vi "KB-SplitRoi TO Recntage.vi"(11 "String 2":string) -> (3 "数组":string[](array[string]))   [LabVIEW 2015]
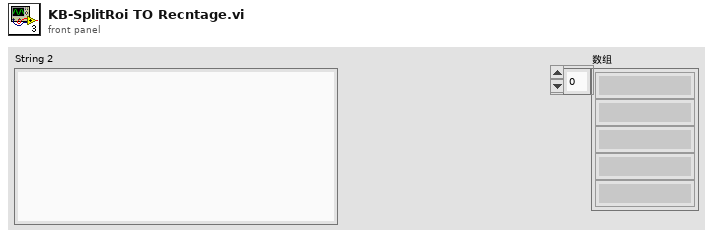
[diagram p1: front panel]
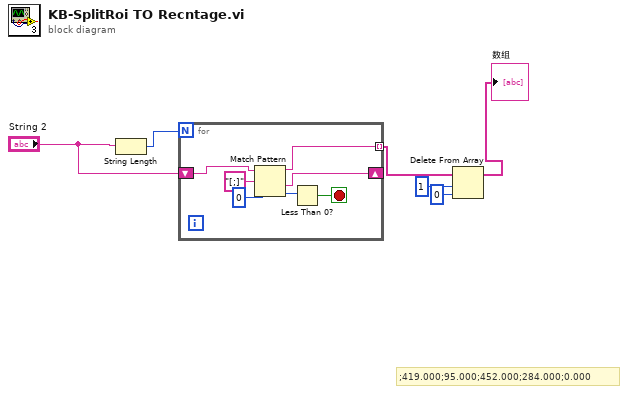
[diagram p0: block diagram]
diagram:
  # ";419.000;95.000;452.000;284.000;0.000"
  n1 = String Length(string="String 2") -> (length=w6:i32)
  n2 = for {
    N: w6 -> [_]
    shift-right: [w8] -> _
    shift-left: "String 2" -> [w9]
    tunnel: [w7] -> w5 mode=indexing
    stop <- w10 stop-if-true
    n3 = Match Pattern(string=w9, regular expression="[;]" ("正则表达式"), offset (0)=0 ("偏移量(0)")) -> (before substring=w7:string, after substring=w8:string, offset past match=w11:i32)  [unwired: 1 out]
    n4 = Less Than 0?(x=w11) -> (x < 0?=w10:bool)
  }
  n5 = Delete From Array(array=w5, length=1 ("长度"), index=0 ("索引")) -> (array with subset deleted=→"数组":string[])  [unwired: 1 out]
